vi "read standards data.vi"() -> (0 "standard cluster array":T1 {"Absorbance" format="%.2e"; "Concentrations" format="%.3e"; "Setup"."sample type" items=["Sample Cuvet", "Sipper Cell", "No Dialog"]; "Setup"."sample time" min=0.0 max=100.0 step=1.0 format="%.1f"; "Setup"."rinse time" min=0.0 max=100.0 step=1.0 format="%.1f"; "Setup"."integration time" format="%.1f"}, 3 "standards array":T4=[{"Standard Description"="Nitrate (molar)", "standards setup"={"integration time"=0.0, "rinse time"=0.0, "sample time"=0.0, "sample type"=0}, "Standard C"=[0.0, 1e-05, 3e-05, 0.0001, 0.0003, 0.001], "extinction"=array[316 elements], "Your name"="Monroe Weber-Shirk", "correlation coef"=[], "units"=""}, {"Standard Description"="Methylene Blue (molar)", "standards setup"={"integration time"=0.0, "rinse time"=0.0, "sample time"=0.0, "sample type"=0}, "Standard C"=[0.0, 1e-05, 3e-05, 0.0001, 0.0003, 0.001], "extinction"=array[316 elements], "Your name"="Monroe Weber-Shirk", "correlation coef"=[], "units"=""}, {"Standard Description"="Nitrate (molar)", "standards setup"={"integration time"=0.0, "rinse time"=0.0, "sample time"=0.0, "sample type"=0}, "Standard C"=[0.0, 1e-05, 3e-05, 0.0001, 0.0003, 0.001], "extinction"=[6e-05, 0.00221, 0.00306, 0.00317, 0.00265, 0.00207, 0.00119, 0.00025, -0.00096, -0.00199, -0.00326, -0.00411, -0.00514, -0.00601, -0.00637, -0.00648, -0.00656, -0.00639, -0.00598, -0.00572, -0.00506, -0.00451, -0.00396, -0.0035, -0.00303, -0.00267, -0.00244, -0.00225, -0.00195, -0.00143, -0.00079, 3e-05, 0.0008, 0.00166, 0.00238, 0.00297, 0.00341, 0.00378, 0.0039, 0.00392, 0.00384, 0.00372, 0.00352, 0.00314, 0.00282, 0.00242, 0.00177, 0.00137, 0.00077, -1e-05, -0.00059, -0.00108, -0.00134, -0.00131, -0.00105, -0.00088, -0.00057, -0.00032, -0.00022, -0.00033, -0.00038, -0.00019, -0.00021, -0.00013, -0.00021, -0.00012, -0.00018, -6e-05, -0.00015, -0.00013, -7e-05, -1e-05, 4e-05, 0.00028, 0.00035, 0.00048, 0.00077, 0.0008, 0.00097, 0.00123, 0.00125, 0.00146, 0.00151, 0.00158, 0.00175, 0.00189, 0.00192, 0.00209, 0.00259, 0.00344, 0.00344, 0.00314, 0.00273, 0.00338, 0.00329, 0.00483, 0.00416, 0.00453, 0.00415, 0.0057, 0.00456, 0.00387, 0.00733, 0.00433, 0.00578, 0.00793, 0.00433, 0.00503, 0.00907, 0.00512, 0.00527, 0.00619, 0.00883, 0.00532, 0.00614, 0.00546, 0.01057, 0.01022, 0.00575, 0.00856, 0.01062, 0.01115, 0.00621, 0.00558, 0.00915, 0.00848, 0.00535, 0.00787, 0.00842, 0.00877, 0.00704, 0.00596, 0.00531, 0.00262, 0.00599, 0.00656, 0.00518, 0.00746, 0.01216, 0.0121, 0.00685, 0.00506, 0.0082, 0.00939, 0.00521, 0.00415, 0.00613, 0.00923, 0.00846, 0.01092, 0.01307, 0.00959, 0.0108, 0.01184, 0.01274, 0.00772, 0.01136, 0.01332, 0.00874, 0.0079, 0.0115, 0.01463, 0.01071, 0.00805, 0.01184, 0.0133, 0.01077, 0.00883, 0.01077, 0.00929, 0.009, 0.00866, 0.00807, 0.00978, 0.01129, 0.00897, 0.00906, 0.0057, 0.01086, 0.01492, 0.0093, 0.00859, 0.01165, 0.01368, 0.01042, 0.00794, 0.0093, 0.00512, -0.00669, -0.0079, -0.00685, 0.00434, -0.00195, 0.00642, 0.00312, 0.00416, -0.00061, -0.00059, -0.0019, -0.00566, -0.00833, 0.00254, 0.0, -0.00189, 0.00862, 0.00765, 0.00112, -0.00064, 0.0028, 0.00683, 0.00155, -0.0003, 0.0054, 0.00462, -0.00639, 0.00265, 0.00604, -0.00057, -0.00447, 0.00471, -0.00041, -0.01329, -0.00877, -0.0001, 0.0025, -0.01448, -0.01643, -0.01341, -0.0164, -0.00784, 0.00132, -0.00469, -0.00727, -0.00599, -0.00289, -0.0079, -0.00978, -0.00033, -0.0065, -0.01058, 0.00389, 0.00607, -0.00247, 0.00625, 0.00309, 0.0075, 0.00675, 0.00238, 0.02153, 0.00531, 0.00671, 0.01777, 0.00942, 0.01489, 0.02458, 0.00833, 0.00894, 0.0129, 0.01617, 0.02844, 0.01483, 0.01608, 0.02296, 0.01797, 0.01881, 0.0142, 0.00575, 0.00914, 0.01087, 0.01379, 0.01463, 0.0223, 0.00849, 0.01046, 0.00225, 0.01255, 0.00628, 0.00013, -0.01025, -0.00317, -0.00169, -0.00013, 0.014, 0.00627, 0.02648, 0.01156, 0.01533, 0.0162, 0.012, 0.00538, 0.01255, -0.00395, -0.00947, -0.0081, -0.0059, -0.00109, 0.01068, 0.00973, 0.0028, 0.00073, 0.01567, 0.01887, 0.02369, 0.02372, 0.01115, 0.01058, 0.00817, 0.00433, 0.00431, 0.01495, -0.00257, 0.00178, -0.00054, 0.00404, 0.01396, 0.00617], "Your name"="Monroe Weber-Shirk", "correlation coef"=[], "units"=""}] {"correlation coef" format="%.3f"; "extinction" format="%.2e"; "Standard C" format="%^.2e"; "standards setup"."sample type" items=["Sample Cuvet", "Sipper Cell", "No Dialog"]; "standards setup"."sample time" min=0.0 max=100.0 step=1.0 format="%.1f"; "standards setup"."rinse time" min=0.0 max=100.0 step=1.0 format="%.1f"; "standards setup"."integration time" format="%.1f"})   [LabVIEW 2015]
uses:
  standards array.ctl
  settings.ctl
  standard cluster array.ctl
  standard cluster.ctl
  <vilib>/Analysis/NI_AALPro.lvlib
  <vilib>/gmath/NI_Gmath.lvlib
panel:
  out "Waveform Graph":dbl[][](graph)
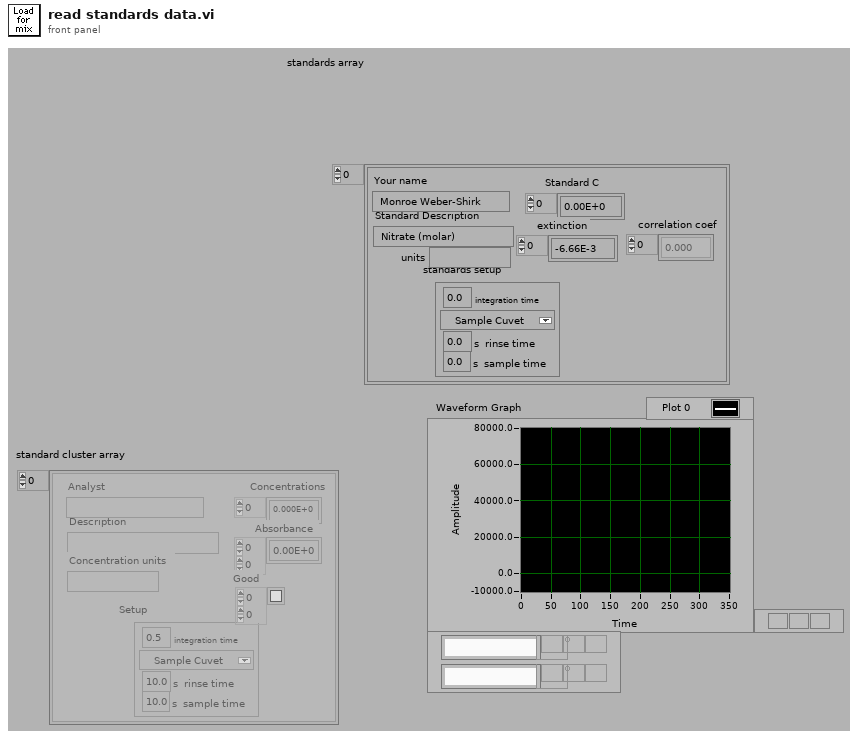
[diagram p1: front panel]
types:
  T1 = typedef "standard cluster array.ctl" = T2[]
  T2 = typedef "standard cluster.ctl" = cluster{"Description":string, "Setup":T3, "Concentrations":dbl[], "Absorbance":dbl[][], "Analyst":string, "Concentration units":string, "Good":bool[][]}
  T3 = typedef "settings.ctl" = cluster{"integration time":sgl, "rinse time":dbl[unit], "sample time":dbl[unit], "sample type":u16}
  T4 = typedef "standards array.ctl" = cluster{"Standard Description":string, "standards setup":T3, "Standard C":dbl[], "extinction":dbl[], "Your name":string, "correlation coef":dbl[], "units":string}[]
  T5 = enum32{"existing file", "new file", "new or existing file", "existing dir", "new dir", "new or existing dir", "existing file (use LLBs)", "new file (use LLBs)", "new or existing file (use LLBs)", "new or existing file or directory (use LLBs)"}
  T6 = cluster{"Standard Description":string, "standards setup":T3, "Standard C":dbl[], "extinction":dbl[], "Your name":string, "correlation coef":dbl[], "units":string}
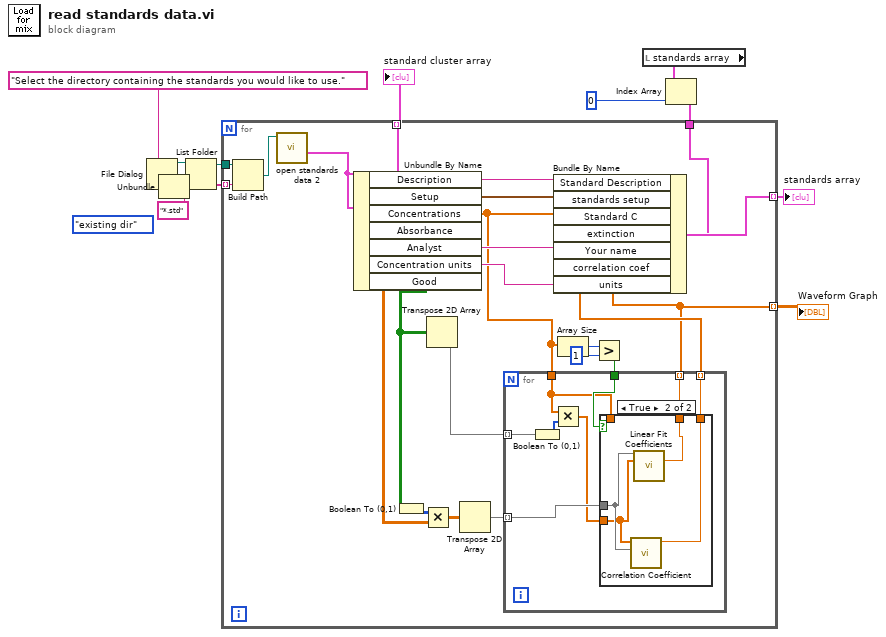
[diagram p0: block diagram]
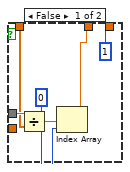
[diagram p2: hidden frame]
diagram:
  (unwired) T5."existing dir" ("select mode (2)")
  n1 = File Dialog(7:"Select the directory containing the standards you would like to use.") -> (0:w1:errorcluster, 3:w11:path)  [unwired: 6 in, 2 out]
  n2 = Unbundle(w1) -> ()  [unwired: 3 out]
  n3 = List Folder(path=w11, pattern="*.std") -> (path out=w9:path, filenames=w10:string[])  [unwired: 2 in, 2 out]
  n4 = local read "standards array"() -> (w4:T4)
  n5 = Index Array(array=w4, index=0 ("Index")) -> (element=w5:T6)
  n6 = for {
    tunnel: w10 -> [w34] mode=indexing
    tunnel: w9 -> [w19]
    tunnel: [w33] -> w8 mode=indexing
    tunnel: [w20] -> w7 mode=indexing
    tunnel: w5 -> [w21]
    tunnel: [w13] -> w2 mode=indexing
    n7 = Build Path(base path=w19, name or relative path=w34) -> (appended path=w18:path)
    n8 = call "open standards data 2.vi"("file path"=w18) -> ("standard cluster"=w20:T2)  [unwired: 8 in, 2 out]
    n9 = Unbundle By Name(w20) -> ("Description"=w32:string, "Setup"=w31:T3, "Concentrations"=w17:dbl[], "Absorbance"=w27:dbl[][], "Analyst"=w30:string, "Concentration units"=w22:string, "Good"=w25:bool[][])
    n10 = Boolean To (0,1)(Boolean=w25) -> (0, 1=w26:i16[][])
    n11 = Multiply(x=w26, y=w27) -> (x*y=w23:dbl[][])
    n12 = Transpose 2D Array(2D array=w25) -> (transposed array=w28:bool[][])
    n13 = Transpose 2D Array(2D array=w23) -> (transposed array=w29:dbl[][])
    n14 = Array Size(array=w17) -> (size(s)=w16:i32)
    n15 = Greater?(x=w16, y=1) -> (0:w14:bool)
    n16 = for {
      tunnel: w29 -> [w37] mode=indexing
      tunnel: [w42] -> w13 mode=indexing
      tunnel: w28 -> [w38] mode=indexing
      tunnel: w17 -> [w35]
      tunnel: [w41] -> w24 mode=indexing
      tunnel: w14 -> [w40]
      n17 = Boolean To (0,1)(Boolean=w38) -> (0, 1=w39:i16[])
      n18 = Multiply(x=w35, y=w39) -> (x*y=w36:dbl[])
      n19 = case shown="True" w40 {
        tunnel: [w45 w49] -> w42
        tunnel: [1 ("index") w52] -> w41
        tunnel: w36 -> [_ w50]
        tunnel: w37 -> [w48 w51]
        tunnel: w35 -> [w43 _]
        frame False {
          n20 = Divide(x=w48, y=w43) -> (x/y=w46:dbl[])
          n21 = Index Array(array=w46, index=0) -> (element=w45:dbl)
        }
        frame True {
          n22 = call <vilib>:"Correlation Coefficient.vi"("Y"=w51, "X"=w50) -> ("correlation coefficient r"=w52:dbl)  [unwired: 8 in, 1 out]
          n23 = call <vilib>:"Linear Fit Coefficients.vi"("Y"=w51, "X"=w50) -> ("intercept"=w49:dbl)  [unwired: 11 in, 2 out]
        }
      }
    }
    n24 = Bundle By Name(cluster=w21, "Standard Description"=w32, "standards setup"=w31, "Standard C"=w17, "extinction"=w13, "Your name"=w30, "correlation coef"=w24, "units"=w22) -> (w33:T6)
  }
  "standards array" <- w8
  "standard cluster array" <- w7
  "Waveform Graph" <- w2
